vi "Cluster type def.vi"() -> ()   [LabVIEW 2020]
uses:
  Cluster def.ctl
panel:
  in  "Cluster 2":T1
  out "String":string
  out "Boolean":bool
  out "Numeric":dbl
  in  "Cluster":T1
  # "Cluster type def"
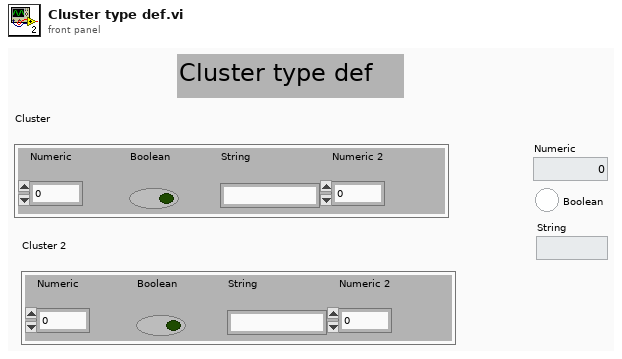
[diagram p1: front panel]
types:
  T1 = typedef "Cluster def.ctl" = cluster{"Numeric":dbl, "Boolean":bool, "String":string, "Numeric 2":dbl}
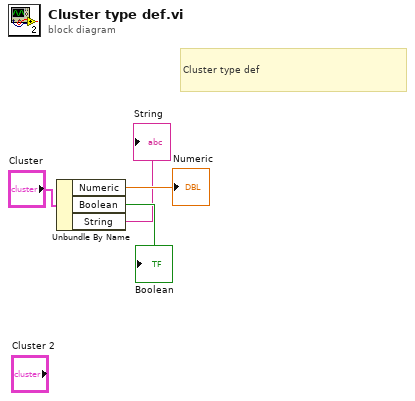
[diagram p0: block diagram]
diagram:
  # "Cluster type def"
  n1 = Unbundle By Name "Unbundle By Name"("Cluster") -> ("Numeric"=→"Numeric":dbl, "Boolean"=→"Boolean":bool, "String"=→"String":string)
